vi "ContinuousCapture.vi"(8 "error in (no error)":errorcluster, 11 "Instruments in":refnum<class "Instruments.lvclass">) -> (0 "error out":errorcluster, 3 "Instruments out":refnum<class "Instruments.lvclass">)   [LabVIEW 2012, in "Instruments.lvclass"]
uses:
  Instruments.lvclass
  Instruments.lvclass/Instruments.ctl
  SpectrumCommands.ctl
  SpectrumWindowExit.vi
  Controls/Config.ctl
panel:
  out "Ready":bool
  in  "Int Time(ms)":i32
  in  "Enabled":bool
  in  "Exit":bool
  in  "StopCapture":bool
  in  "StartCapture":bool
  in  "Graph":cluster{"Y":dbl[], "Y":dbl[]}[](graph)
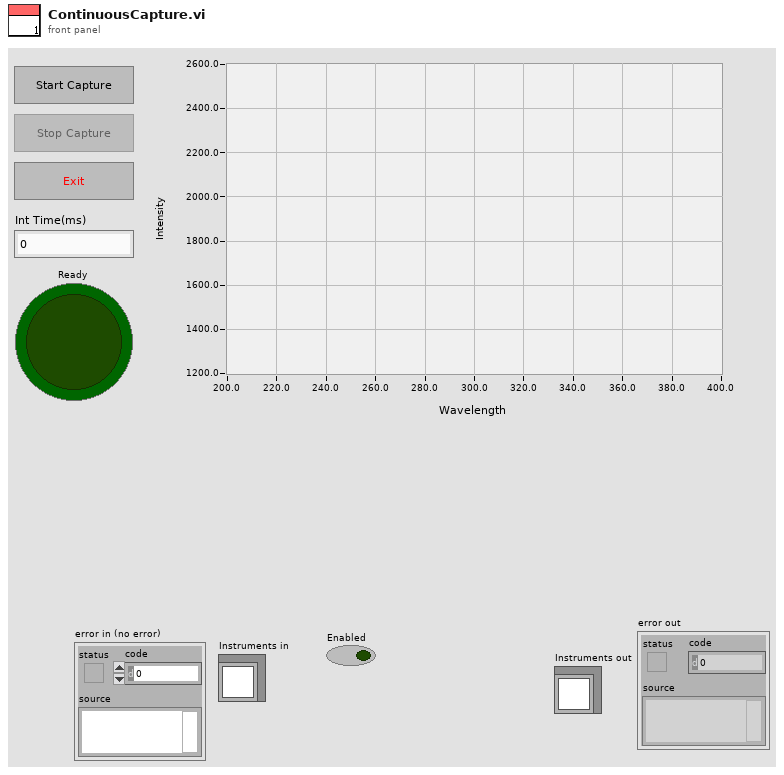
[diagram p1: front panel]
types:
  T1 = enum8{"Enabled", "Disabled", "Disabled and Grayed Out"}
  T2 = cluster{"StopCapture":refnum<vi>, "StartCapture":refnum<vi>, "Exit":refnum<vi>, "Enabled":refnum<vi>, "Ready":refnum<vi>}
  T3 = typedef "Config.ctl" = cluster{"IntTime":i32, "Samples":i32, "PowerMin":dbl, "KneeMin":dbl, "KneeMax":dbl, "BackgroundWl":dbl}
  T4 = typedef "SpectrumCommands.ctl" = enum16{"Init", "StartCapture", "StopCapture", "Exit"}
  T5 = cluster{"Wavelength":dbl[], "EL Spectrum":dbl[]}[]
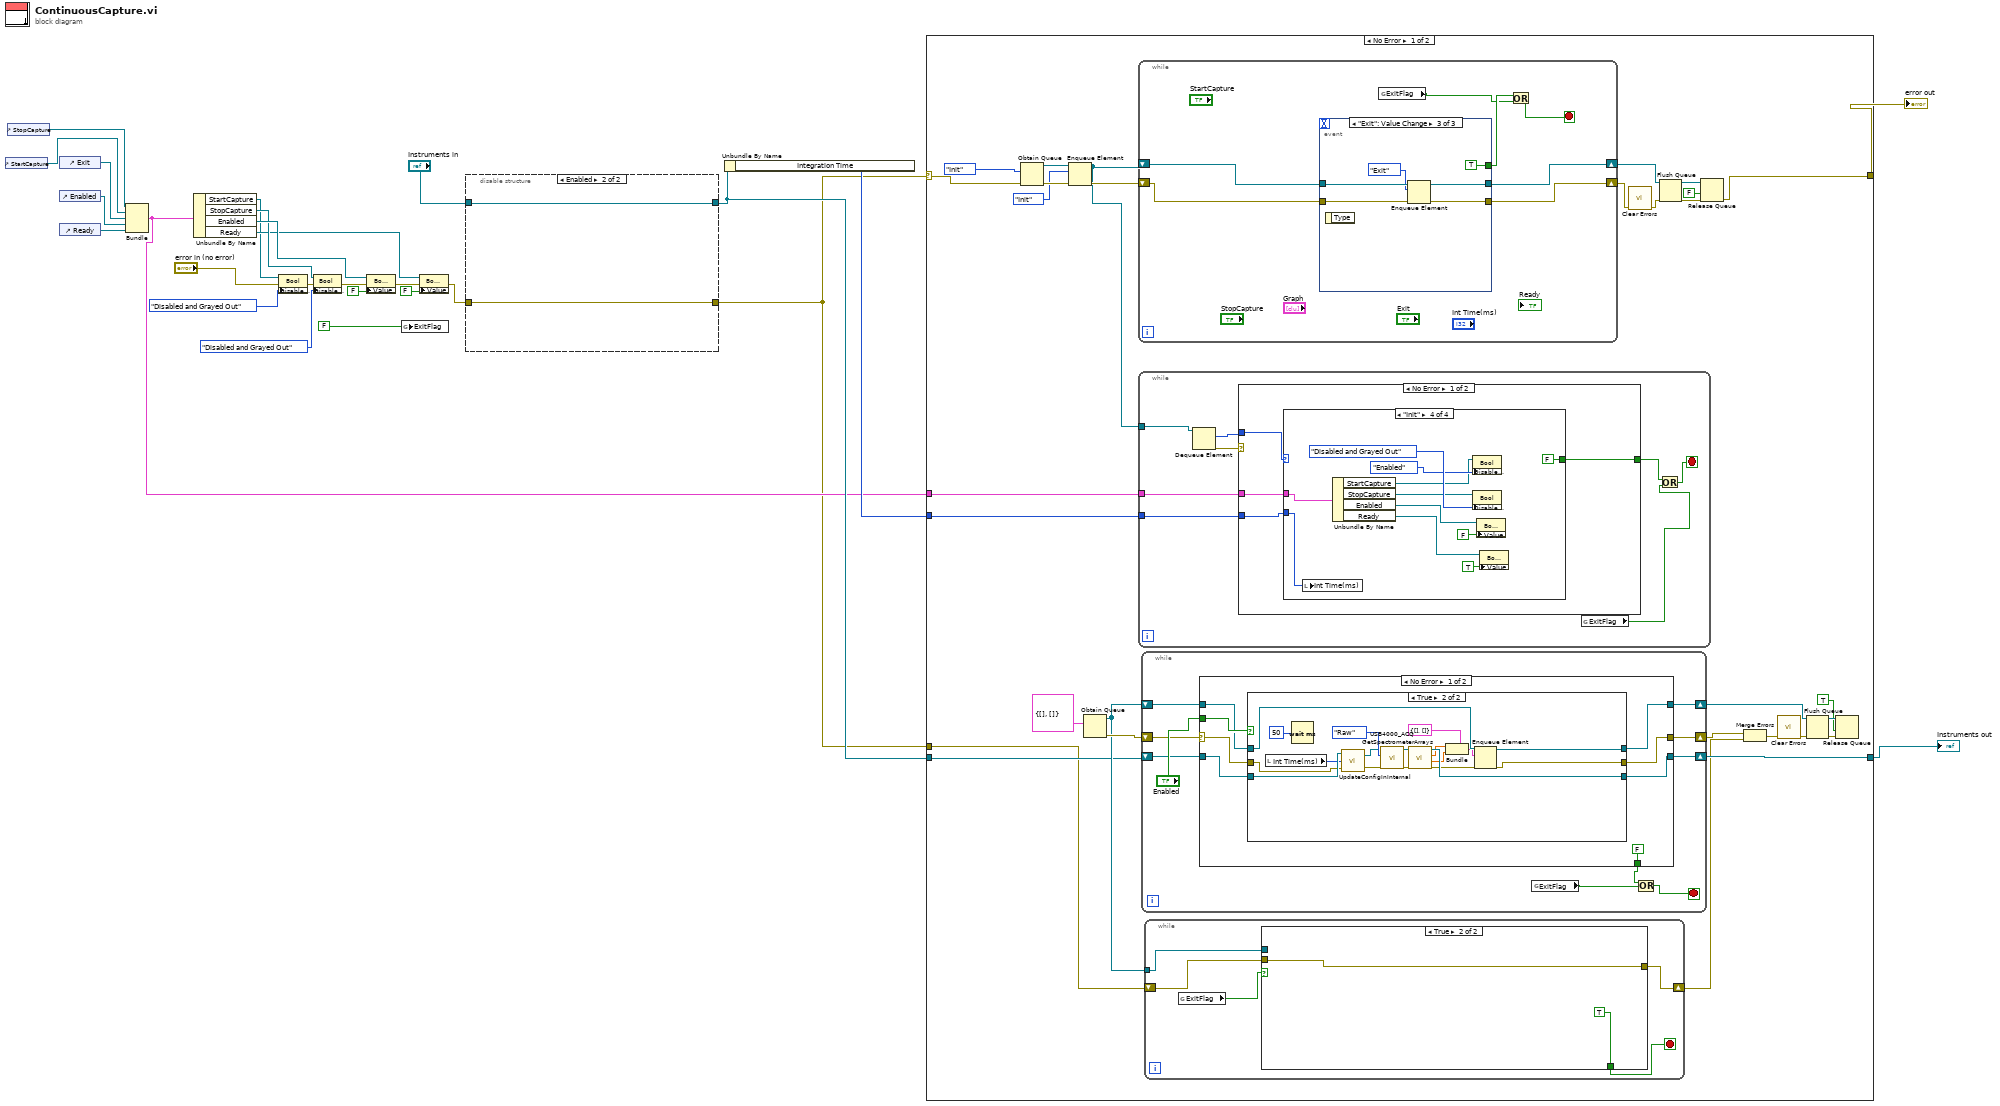
[diagram p0: block diagram]
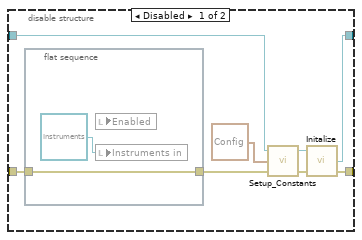
[diagram p2: hidden frame]
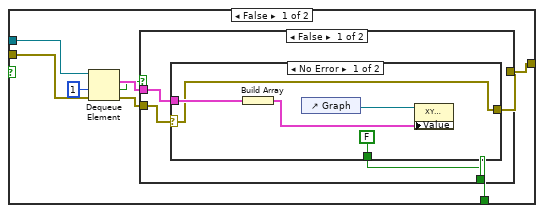
[diagram p3: hidden frame]
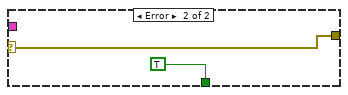
[diagram p4: hidden frame]
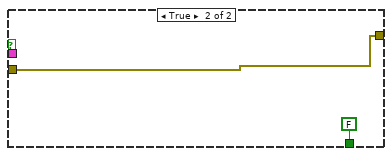
[diagram p5: hidden frame]
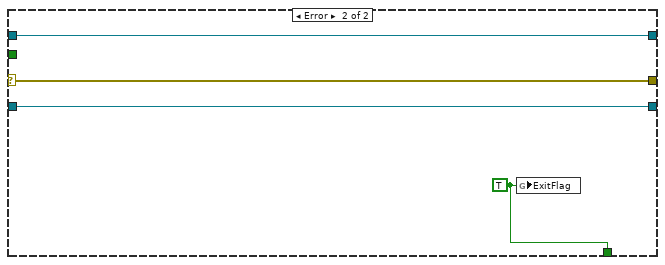
[diagram p7: hidden frame]
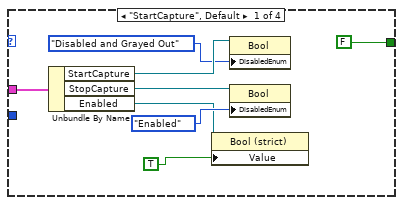
[diagram p8: hidden frame]
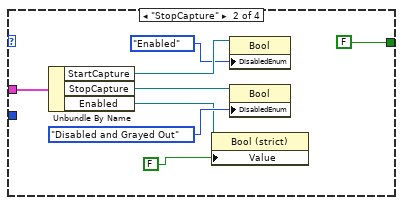
[diagram p9: hidden frame]
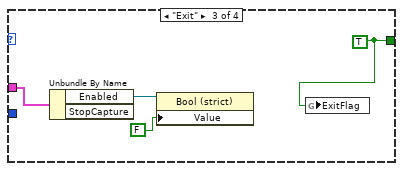
[diagram p10: hidden frame]
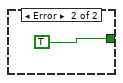
[diagram p11: hidden frame]
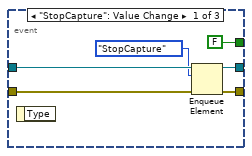
[diagram p12: hidden frame]
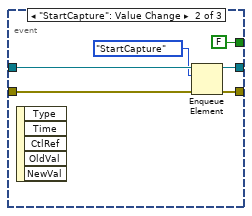
[diagram p13: hidden frame]
diagram:
  n1 = control-ref of="StartCapture"() -> (w23:refnum<vi>)
  n2 = control-ref of="StopCapture"() -> (w24:refnum<vi>)
  n3 = control-ref of="Exit"() -> (w22:refnum<vi>)
  n4 = control-ref of="Enabled"() -> (w21:refnum<vi>)
  n5 = control-ref of="Ready"() -> (w17:refnum<vi>)
  n6 = Bundle("StopCapture"=w24, "StartCapture"=w23, "Exit"=w22, "Enabled"=w21, "Ready"=w17) -> (w4:T2)  [unwired: 1 in]
  n7 = Unbundle By Name(w4) -> ("StartCapture"=w9:refnum<vi>, "StopCapture"=w13:refnum<vi>, "Enabled"=w15:refnum<vi>, "Ready"=w11:refnum<vi>)
  n8 = property class="Bool"(reference=w9, error in="error in (no error)", "DisabledEnum"=T1."Disabled and Grayed Out" ("Disabled")) -> (error out=w7:errorcluster)  [unwired: 1 out]
  n9 = property class="Bool"(reference=w13, error in=w7, "DisabledEnum"=T1."Disabled and Grayed Out" ("Disabled")) -> (error out=w6:errorcluster)  [unwired: 1 out]
  n10 = property class="Bool (strict)"(reference=w15, error in=w6, "Value"=FALSE) -> (error out=w5:errorcluster)  [unwired: 1 out]
  n11 = global write "SpectrumWindowExit.vi" "ExitFlag"(FALSE ("Enabled")) -> ()
  n12 = property class="Bool (strict)"(reference=w11, error in=w5, "Value"=FALSE) -> (error out=w3:errorcluster)  [unwired: 1 out]
  n13 = disable-structure shown="Enabled" {
    disable-tunnel: [w34 w37] -> w19
    disable-tunnel: [w33 w38] -> w2
    disable-tunnel: "Instruments in" -> [w29 w37]
    disable-tunnel: w3 -> [w27 w38]
    frame Disabled {
      n14 = flat-sequence {
        tunnel: [w35] -> w28
        tunnel: w27 -> [w35]
        frame #0 {
          n15 = local read "Enabled"() -> ()  [unwired: 1 in]
          n16 = local write "Instruments in"(refnum<class "Instruments.lvclass"> refnum ("Instruments in")) -> ()
        }
      }
      n17 = call-dynamic "Setup_Constants.vi"("error in (no error)"=w28, "Config In"=T3 {"IntTime"=100, "Samples"=3, "PowerMin"=300.0, "KneeMin"=-20.0, "KneeMax"=20.0, "BackgroundWl"=275.0}, "Instruments in"=w29) -> ("error out"=w30:errorcluster, "Instruments out"=w31:refnum<class "Instruments.lvclass">)  [unwired: 1 in]
      n18 = call-dynamic "Initalize.vi"("error in (no error)"=w30, "Instruments in"=w31) -> ("error out"=w33:errorcluster, "Instruments out"=w34:refnum<class "Instruments.lvclass">)  [unwired: 2 in]
    }
    frame Enabled {
    }
  }
  n19 = Unbundle By Name(w19) -> ("Integration Time"=w18:i32)
  n20 = case shown="No Error" w2 {
    selector: w2 -> [w67 w210]
    tunnel: [w57 w210] -> w26
    tunnel: [w64 w209] -> w25
    tunnel: w19 -> [w62 w209]
    tunnel: w4 -> [w39 _]
    tunnel: w2 -> [w61 _]
    tunnel: w18 -> [w41 _]
    frame No Error {
      n21 = Obtain Queue(element data type=SpectrumCommands."Init", error in (no error)=w67) -> (queue out=w45:refnum<queue>, error out=w44:errorcluster)  [unwired: 3 in, 1 out]
      n22 = Enqueue Element(queue=w45, element=SpectrumCommands."Init", error in (no error)=w44) -> (queue out=w40:refnum<queue>, error out=w42:errorcluster)  [unwired: 1 in, 1 out]
      n23 = Obtain Queue(element data type=cluster{"Wavelength":dbl[], "EL Spectrum":dbl[]} {"Wavelength"=[], "EL Spectrum"=[]}) -> (queue out=w63:refnum<queue>, error out=w65:errorcluster)  [unwired: 4 in, 1 out]
      n24 = while {
        shift-right: [w187] -> w58
        shift-left: w40 -> [w190]
        shift-right: [w188] -> w51
        shift-left: w42 -> [w189]
        stop <- w185 stop-if-true
        n25 = event shown="[2] \"Exit\": Value Change" {
          selector: _ -> [_ _ _]
          dyn-events: _ -> [_ _ _]
          timeout: _ -> [_ _ _]
          tunnel: w190 -> [w196 w202 w208]
          tunnel: w189 -> [w195 w201 w207]
          tunnel: [w194 w200 w206] -> w188
          tunnel: [w193 w199 w205] -> w187
          tunnel: [FALSE ("ExitFlag") FALSE ("ExitFlag") TRUE ("ExitFlag")] -> w186
          event "StopCapture": Value Change {
            n26 = event-data() -> ()  [unwired: 1 in, 1 out]
            n27 = Enqueue Element(queue=w196, element=SpectrumCommands."StopCapture", error in (no error)=w195) -> (queue out=w193:refnum<queue>, error out=w194:errorcluster)  [unwired: 1 in, 1 out]
          }
          event "StartCapture": Value Change {
            n28 = event-data() -> ()  [unwired: 1 in, 5 out]
            n29 = Enqueue Element(queue=w202, element=SpectrumCommands."StartCapture", error in (no error)=w201) -> (queue out=w199:refnum<queue>, error out=w200:errorcluster)  [unwired: 1 in, 1 out]
          }
          event "Exit": Value Change {
            n30 = event-data() -> ()  [unwired: 1 in, 1 out]
            n31 = Enqueue Element(queue=w208, element=SpectrumCommands."Exit", error in (no error)=w207) -> (queue out=w205:refnum<queue>, error out=w206:errorcluster)  [unwired: 1 in, 1 out]
          }
        }
        n32 = global read "SpectrumWindowExit.vi" "ExitFlag"() -> (w184:bool)
        n33 = Or(x=w186, y=w184) -> (x .or. y?=w185:bool)
      }
      n34 = while {
        tunnel: w39 -> [w145]
        tunnel: w41 -> [w141]
        tunnel: w40 -> [w140]
        stop <- w143 stop-if-true
        n35 = Dequeue Element(queue=w140) -> (element=w146:T4, error out=w147:errorcluster)  [unwired: 2 in, 2 out]
        n36 = case shown="No Error" w147 {
          tunnel: w146 -> [w151 _]
          tunnel: w145 -> [w150 _]
          tunnel: [w149 TRUE ("x")] -> w144
          tunnel: w141 -> [w148 _]
          frame No Error {
            n37 = case shown="\"Init\"" w151 {
              tunnel: w150 -> [w159 w162 w171 w175]
              tunnel: [FALSE ("x") FALSE ("x") w168 FALSE ("x")] -> w149
              tunnel: w148 -> [_ _ _ w181]
              frame "StartCapture", Default {
                n38 = Unbundle By Name(w159) -> ("StartCapture"=w158:refnum<vi>, "StopCapture"=w156:refnum<vi>, "Enabled"=w154:refnum<vi>)
                n39 = property class="Bool (strict)"(reference=w154, "Value"=TRUE) -> ()  [unwired: 1 in, 2 out]
                n40 = property class="Bool"(reference=w158, "DisabledEnum"=T1."Disabled and Grayed Out" ("Disabled")) -> ()  [unwired: 1 in, 2 out]
                n41 = property class="Bool"(reference=w156, "DisabledEnum"=T1."Enabled" ("Disabled")) -> ()  [unwired: 1 in, 2 out]
              }
              frame "StopCapture" {
                n42 = Unbundle By Name(w162) -> ("StartCapture"=w167:refnum<vi>, "StopCapture"=w165:refnum<vi>, "Enabled"=w163:refnum<vi>)
                n43 = property class="Bool (strict)"(reference=w163, "Value"=FALSE) -> ()  [unwired: 1 in, 2 out]
                n44 = property class="Bool"(reference=w167, "DisabledEnum"=T1."Enabled" ("Disabled")) -> ()  [unwired: 1 in, 2 out]
                n45 = property class="Bool"(reference=w165, "DisabledEnum"=T1."Disabled and Grayed Out" ("Disabled")) -> ()  [unwired: 1 in, 2 out]
              }
              frame "Exit" {
                w168 = TRUE ("x")
                n46 = Unbundle By Name(w171) -> ("Enabled"=w170:refnum<vi>)  [unwired: 1 out]
                n47 = property class="Bool (strict)"(reference=w170, "Value"=FALSE) -> ()  [unwired: 1 in, 2 out]
                n48 = global write "SpectrumWindowExit.vi" "ExitFlag"(w168) -> ()
              }
              frame "Init" {
                n49 = local write "Int Time(ms)"(w181) -> ()
                n50 = Unbundle By Name(w175) -> ("StartCapture"=w172:refnum<vi>, "StopCapture"=w177:refnum<vi>, "Enabled"=w179:refnum<vi>, "Ready"=w174:refnum<vi>)
                n51 = property class="Bool"(reference=w172, "DisabledEnum"=T1."Enabled" ("Disabled")) -> ()  [unwired: 1 in, 2 out]
                n52 = property class="Bool"(reference=w177, "DisabledEnum"=T1."Disabled and Grayed Out" ("Disabled")) -> ()  [unwired: 1 in, 2 out]
                n53 = property class="Bool (strict)"(reference=w179, "Value"=FALSE) -> ()  [unwired: 1 in, 2 out]
                n54 = property class="Bool (strict)"(reference=w174, "Value"=TRUE) -> ()  [unwired: 1 in, 2 out]
              }
            }
          }
          frame Error {
          }
        }
        n55 = global read "SpectrumWindowExit.vi" "ExitFlag"() -> (w142:bool)
        n56 = Or(x=w144, y=w142) -> (x .or. y?=w143:bool)
      }
      n57 = while {
        shift-right: [w102] -> w52
        shift-left: w63 -> [w103]
        shift-right: [w104] -> w64
        shift-left: w62 -> [w105]
        shift-right: [w101] -> w49
        shift-left: w65 -> [w100]
        stop <- w99 stop-if-true
        n58 = case shown="No Error" w100 {
          selector: w100 -> [w108 w137]
          tunnel: "Enabled" -> [w114 _]
          tunnel: w105 -> [w113 w138]
          tunnel: [w112 w138] -> w104
          tunnel: w103 -> [w111 w139]
          tunnel: [w110 w139] -> w102
          tunnel: [w109 w137] -> w101
          tunnel: [FALSE ("ExitFlag") w136] -> w98
          frame No Error {
            n59 = case shown="True" w114 {
              tunnel: w113 -> [w116 w122]
              tunnel: [w116 w130] -> w112
              tunnel: w111 -> [w117 w133]
              tunnel: [w117 w131] -> w110
              tunnel: [w115 w128] -> w109
              tunnel: w108 -> [w115 w120]
              frame False {
              }
              frame True {
                n60 = local read "Int Time(ms)"() -> (w121:i32)
                n61 = Wait (ms)(milliseconds to wait=u32 50) -> ()  [unwired: 1 out]
                n62 = call-dynamic "UpdateConfigInInternal.vi"("error in (no error)"=w120, "IntTime"=w121, "Instruments in"=w122) -> ("error out"=w118:errorcluster, "Instruments out"=w119:refnum<class "Instruments.lvclass">)
                n63 = call-dynamic "USB4000_ACQ.vi"("error in (no error)"=w118, "Type"=enum16{"Get Background", "Measure", "Raw"}."Raw", "Instruments in"=w119) -> ("error out"=w134:errorcluster, "Instruments out"=w135:refnum<class "Instruments.lvclass">)  [unwired: 6 in, 1 out]
                n64 = call-dynamic "GetSpectrometerArrays.vi"("error in (no error)"=w134, "Instruments in"=w135) -> ("error out"=w129:errorcluster, "Spectrum"=w123:dbl[], "Wavelength"=w124:dbl[], "Instruments out"=w130:refnum<class "Instruments.lvclass">)  [unwired: 6 in]
                n65 = Bundle(cluster=cluster{"Wavelength":dbl[], "EL Spectrum":dbl[]} {"Wavelength"=[], "EL Spectrum"=[]}, "Wavelength"=w124, "EL Spectrum"=w123) -> (w132:cluster{"Wavelength":dbl[], "EL Spectrum":dbl[]})
                n66 = Enqueue Element(queue=w133, element=w132, error in (no error)=w129) -> (queue out=w131:refnum<queue>, error out=w128:errorcluster)  [unwired: 1 in, 1 out]
              }
            }
          }
          frame Error {
            w136 = TRUE ("ExitFlag")
            n67 = global write "SpectrumWindowExit.vi" "ExitFlag"(w136) -> ()
          }
        }
        n68 = global read "SpectrumWindowExit.vi" "ExitFlag"() -> (w97:bool)
        n69 = Or(x=w98, y=w97) -> (x .or. y?=w99:bool)
      }
      n70 = while {
        tunnel: w63 -> [w69]
        shift-right: [w73] -> w48
        shift-left: w61 -> [w71]
        stop <- w70 stop-if-true
        n71 = global read "SpectrumWindowExit.vi" "ExitFlag"() -> (w72:bool)
        n72 = case shown="True" w72 {
          tunnel: [w79 w96] -> w73
          tunnel: w71 -> [w76 w96]
          tunnel: [w78 TRUE] -> w70
          tunnel: w69 -> [w77 _]
          frame False {
            n73 = Dequeue Element(queue=w77, timeout in ms (-1)=1, error in (no error)=w76) -> (element=w80:cluster{"Wavelength":dbl[], "EL Spectrum":dbl[]}, timed out?=w74:bool, error out=w81:errorcluster)  [unwired: 1 out]
            n74 = case shown="False" w74 {
              tunnel: w81 -> [w85 w94]
              tunnel: w80 -> [w84 _]
              tunnel: [w83 w94] -> w79
              tunnel: [w82 FALSE] -> w78
              frame False {
                n75 = case shown="No Error" w85 {
                  selector: w85 -> [w86 w91]
                  tunnel: w84 -> [w90 _]
                  tunnel: [FALSE TRUE] -> w82
                  tunnel: [w86 w91] -> w83
                  frame No Error {
                    n76 = Build Array(w90) -> (w87:T5)
                    n77 = control-ref of="Graph"() -> (w88:refnum<vi>)
                    n78 = property class="XYGraph (strict)"(reference=w88, "Value"=w87) -> ()  [unwired: 1 in, 2 out]
                  }
                  frame Error {
                  }
                }
              }
              frame True {
              }
            }
          }
          frame True {
          }
        }
      }
      n79 = call <vilib>:"Clear Errors.vi"("error in (no error)"=w51) -> ("error out"=w50:errorcluster)  [unwired: 6 in]
      n80 = Flush Queue(queue=w58, error in (no error)=w50) -> (queue out=w60:refnum<queue>, error out=w59:errorcluster)  [unwired: 1 out]
      n81 = Release Queue(queue=w60, force destroy? (F)=FALSE, error in (no error)=w59) -> (error out=w57:errorcluster)  [unwired: 2 out]
      n82 = Merge Errors(w49, w48) -> (w47:errorcluster)
      n83 = call <vilib>:"Clear Errors.vi"("error in (no error)"=w47) -> ("error out"=w46:errorcluster)  [unwired: 6 in]
      n84 = Flush Queue(queue=w52, error in (no error)=w46) -> (queue out=w55:refnum<queue>, error out=w54:errorcluster)  [unwired: 1 out]
      n85 = Release Queue(queue=w55, force destroy? (F)=TRUE, error in (no error)=w54) -> ()  [unwired: 3 out]
    }
    frame Error {
    }
  }
  "error out" <- w26
  "Instruments out" <- w25
